vi "String Contents.vi"   [LabVIEW 2020]
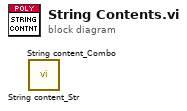
[diagram p0: block diagram]
diagram:
  n1 = call "String content_Str.vi"() -> ()  [unwired: 10 in, 2 out]
  n2 = call "String content_Combo.vi"() -> ()  [unwired: 10 in, 2 out]
